vi "FPGA_Digital Input.vi"(11 "Digital Input":T2={"DI 0"="RMC/DIO15", "DI 1"="RMC/DIO47", "DI 2"="RMC/DIO46", "DI 3"="RMC/DIO79", "DI 4"="RMC/DIO63", "DI 5"="RMC/DIO14", "DI 6"="RMC/DIO78", "DI 7"="RMC/DIO31", "DI 8"="RMC/DIO95", "DI 9"="RMC/DIO13", "DI 10"="RMC/DIO45", "DI 11"="RMC/DIO30"}) -> (3 "Digital Input Data":T1)   [LabVIEW 2018]
uses:
  Data Def/FPGA_Digital Input.ctl
  Data Def/FPGA_Digital Input Data.ctl
  <vilib>/rvi/eio/common/nirviEmuTemplateMethod_errors.vi
  <vilib>/eio/EIONode/EIONode.xnode
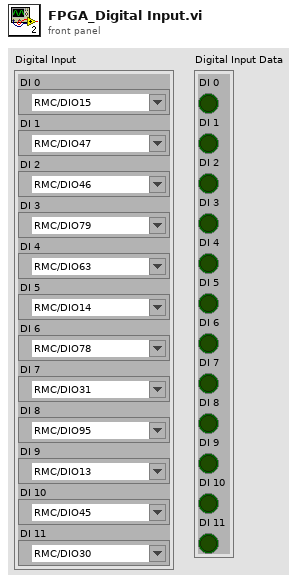
[diagram p1: front panel]
types:
  T1 = typedef "FPGA_Digital Input Data.ctl" = cluster{"DI 0":bool, "DI 1":bool, "DI 2":bool, "DI 3":bool, "DI 4":bool, "DI 5":bool, "DI 6":bool, "DI 7":bool, "DI 8":bool, "DI 9":bool, "DI 10":bool, "DI 11":bool}
  T2 = typedef "FPGA_Digital Input.ctl" = cluster{"DI 0":refnum<k21>, "DI 1":refnum<k21>, "DI 2":refnum<k21>, "DI 3":refnum<k21>, "DI 4":refnum<k21>, "DI 5":refnum<k21>, "DI 6":refnum<k21>, "DI 7":refnum<k21>, "DI 8":refnum<k21>, "DI 9":refnum<k21>, "DI 10":refnum<k21>, "DI 11":refnum<k21>}
  T3 = cluster{"I/O Item":bool, "I/O Item":bool, "I/O Item":bool, "I/O Item":bool, "I/O Item":bool, "I/O Item":bool, "I/O Item":bool, "I/O Item":bool, "I/O Item":bool, "I/O Item":bool, "I/O Item":bool, "I/O Item":bool}
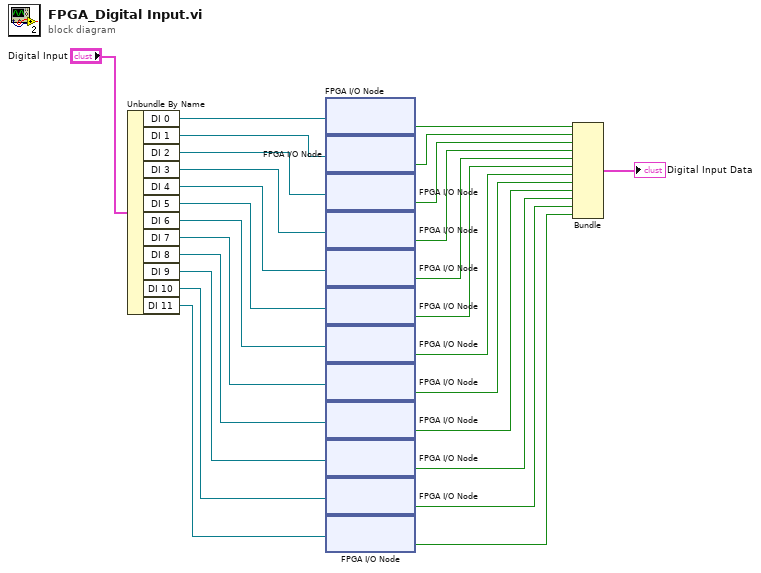
[diagram p0: block diagram]
diagram:
  n1 = Unbundle By Name("Digital Input") -> ("DI 0"=w25:refnum<k21>, "DI 1"=w24:refnum<k21>, "DI 2"=w23:refnum<k21>, "DI 3"=w22:refnum<k21>, "DI 4"=w21:refnum<k21>, "DI 5"=w20:refnum<k21>, "DI 6"=w19:refnum<k21>, "DI 7"=w18:refnum<k21>, "DI 8"=w17:refnum<k21>, "DI 9"=w16:refnum<k21>, "DI 10"=w15:refnum<k21>, "DI 11"=w14:refnum<k21>)
  n2 = xnode "FPGA I/O Node"("FPGA I/O In"=w25) -> ("I/O Item"=w13:bool)  [unwired: 1 out]
  n3 = xnode "FPGA I/O Node"("FPGA I/O In"=w24) -> ("I/O Item"=w12:bool)  [unwired: 1 out]
  n4 = xnode "FPGA I/O Node"("FPGA I/O In"=w23) -> ("I/O Item"=w11:bool)  [unwired: 1 out]
  n5 = xnode "FPGA I/O Node"("FPGA I/O In"=w22) -> ("I/O Item"=w10:bool)  [unwired: 1 out]
  n6 = xnode "FPGA I/O Node"("FPGA I/O In"=w21) -> ("I/O Item"=w9:bool)  [unwired: 1 out]
  n7 = xnode "FPGA I/O Node"("FPGA I/O In"=w20) -> ("I/O Item"=w8:bool)  [unwired: 1 out]
  n8 = xnode "FPGA I/O Node"("FPGA I/O In"=w19) -> ("I/O Item"=w7:bool)  [unwired: 1 out]
  n9 = xnode "FPGA I/O Node"("FPGA I/O In"=w18) -> ("I/O Item"=w6:bool)  [unwired: 1 out]
  n10 = xnode "FPGA I/O Node"("FPGA I/O In"=w17) -> ("I/O Item"=w5:bool)  [unwired: 1 out]
  n11 = xnode "FPGA I/O Node"("FPGA I/O In"=w16) -> ("I/O Item"=w4:bool)  [unwired: 1 out]
  n12 = xnode "FPGA I/O Node"("FPGA I/O In"=w15) -> ("I/O Item"=w3:bool)  [unwired: 1 out]
  n13 = xnode "FPGA I/O Node"("FPGA I/O In"=w14) -> ("I/O Item"=w2:bool)  [unwired: 1 out]
  n14 = Bundle("I/O Item"=w13, "I/O Item"=w12, "I/O Item"=w11, "I/O Item"=w10, "I/O Item"=w9, "I/O Item"=w8, "I/O Item"=w7, "I/O Item"=w6, "I/O Item"=w5, "I/O Item"=w4, "I/O Item"=w3, "I/O Item"=w2) -> (→"Digital Input Data":T3)  [unwired: 1 in]
